vi "Add to data plot.vi"(1 "Data Plot In":T2, 2 "All Data":T1 format="%^_6g", 3 "X-Axis":u32) -> (0 "Data PlotOut":T2)   [LabVIEW 2019]
uses:
  Sub Controls/Data Graph.ctl
  Sub Controls/All Data Array.ctl
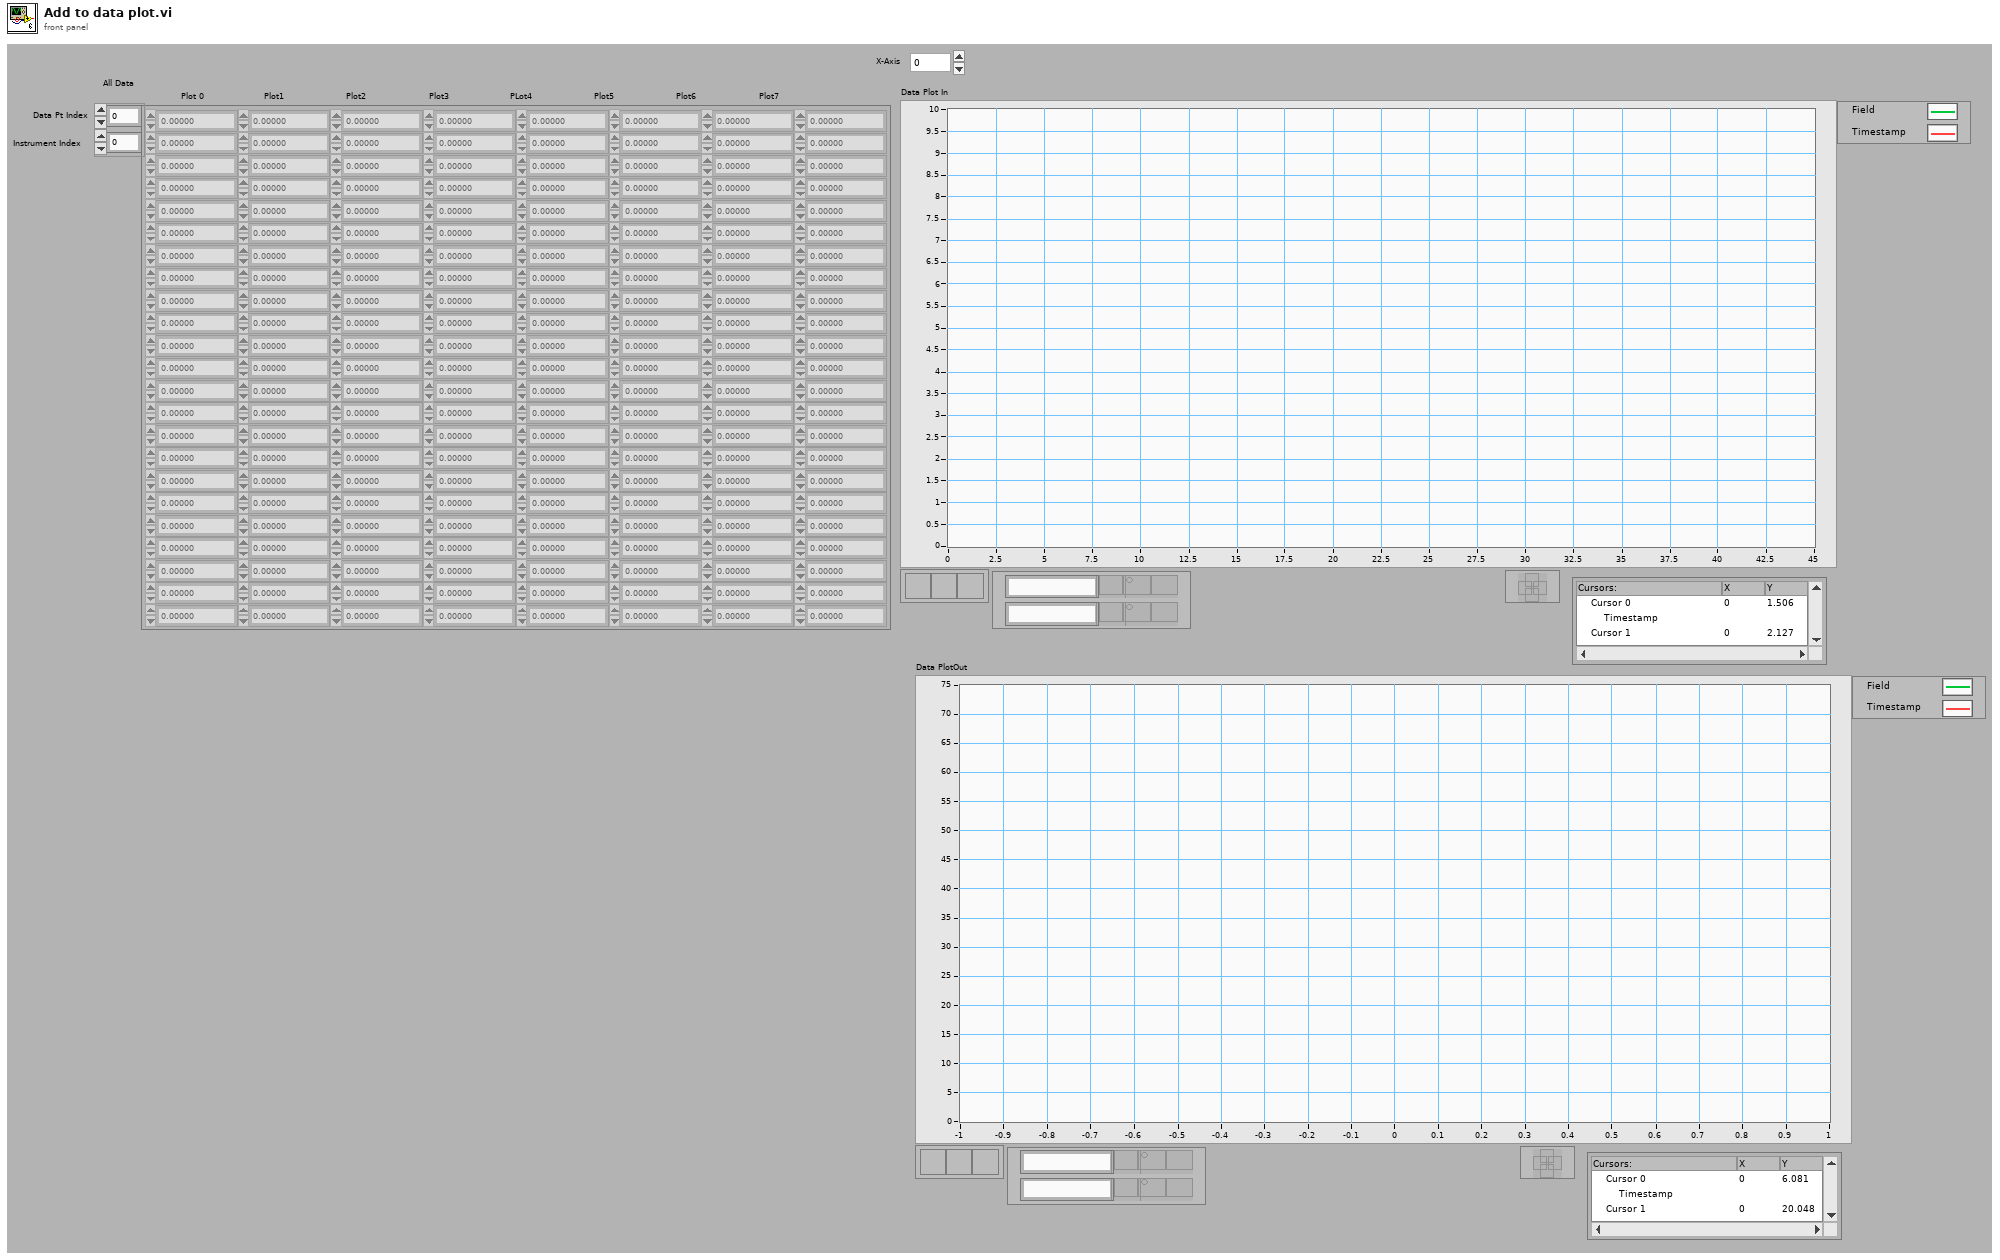
[diagram p1: front panel]
types:
  T1 = typedef "All Data Array.ctl" = dbl[][]
  T2 = typedef "Data Graph.ctl" = cluster{dbl[], dbl[]}[]
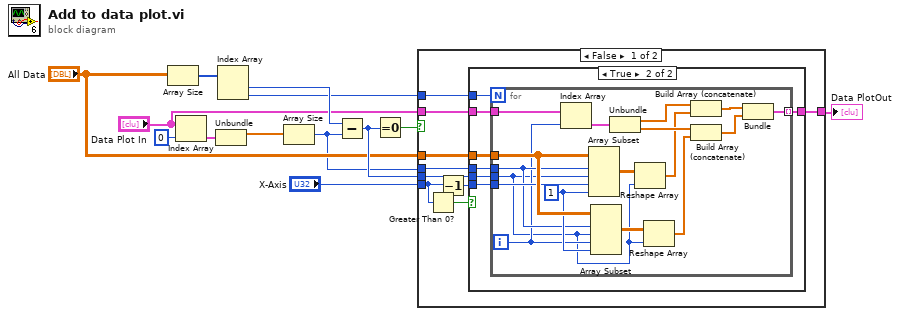
[diagram p0: block diagram]
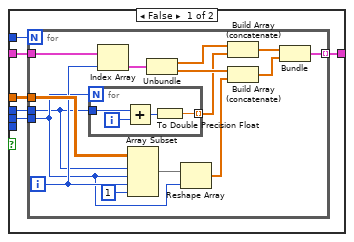
[diagram p2: hidden frame]
diagram:
  n1 = Array Size(array="All Data") -> (size(s)=w10:i32[])
  n2 = Index Array(array="Data Plot In", index=0) -> (element=w9:cluster{dbl[], dbl[]})
  n3 = Unbundle(w9) -> (w8:dbl[])  [unwired: 1 out]
  n4 = Index Array(array=w10) -> (element #1=w11:i32, element #2=w2:i32)  [unwired: 2 in]
  n5 = Array Size(array=w8) -> (size(s)=w4:i32)
  n6 = Subtract(x=w11, y=w4) -> (x-y=w6:i32)
  n7 = Equal To 0?(x=w6) -> (x = 0?=w12:bool)
  n8 = case shown="False" w12 {
    tunnel: [w18 w72] -> w13
    tunnel: "Data Plot In" -> [w22 w72]
    tunnel: w6 -> [w19 _]
    tunnel: "All Data" -> [w21 _]
    tunnel: w4 -> [w20 _]
    tunnel: "X-Axis" -> [w15 _]
    tunnel: w2 -> [w17 _]
    frame False {
      n9 = Greater Than 0?(x=w15) -> (x > 0?=w16:bool)
      n10 = Decrement(x=w15) -> (x-1=w14:u32)
      n11 = case shown="True" w16 {
        tunnel: w22 -> [w23 w54]
        tunnel: w21 -> [w26 w53]
        tunnel: w20 -> [w25 w52]
        tunnel: w19 -> [w24 w51]
        tunnel: [w27 w50] -> w18
        tunnel: w14 -> [_ w49]
        tunnel: w17 -> [w28 w48]
        frame False {
          n12 = for {
            N: w28 -> [_]
            tunnel: w23 -> [w43]
            tunnel: w26 -> [w42]
            tunnel: w25 -> [w30]
            tunnel: w24 -> [w31]
            tunnel: [w40] -> w27 mode=indexing
            i -> [w33]
            n13 = for {
              N: w31 -> [_]
              tunnel: w30 -> [w47]
              tunnel: [w44] -> w29 mode=indexing
              i -> [w46]
              n14 = Add(x=w47, y=w46) -> (x+y=w45:i32)
              n15 = To Double Precision Float(number=w45) -> (double precision float=w44:dbl)
            }
            n16 = Index Array(array=w43, index=w33) -> (element=w34:cluster{dbl[], dbl[]})
            n17 = Array Subset(array=w42, index (row)=w30, length (row)=w31, index (col)=w33, length (col)=1 ("length")) -> (w38:T1)
            n18 = Unbundle(w34) -> (w32:dbl[], w37:dbl[])
            n19 = Reshape Array(w38, w31) -> (w36:dbl[])
            n20 = Build Array (concatenate)(w32, w29) -> (w41:dbl[])
            n21 = Build Array (concatenate)(w37, w36) -> (w39:dbl[])
            n22 = Bundle(w41, w39) -> (w40:cluster{dbl[], dbl[]})  [unwired: 1 in]
          }
        }
        frame True {
          n23 = for {
            N: w48 -> [_]
            tunnel: w54 -> [w71]
            tunnel: w53 -> [w70]
            tunnel: w52 -> [w59]
            tunnel: w51 -> [w55]
            tunnel: [w67] -> w50 mode=indexing
            tunnel: w49 -> [w61]
            i -> [w57]
            w60 = 1 ("length")
            n24 = Index Array(array=w71, index=w57) -> (element=w58:cluster{dbl[], dbl[]})
            n25 = Array Subset(array=w70, index (row)=w59, length (row)=w55, index (col)=w61, length (col)=w60) -> (w69:T1)
            n26 = Array Subset(array=w70, index (row)=w59, length (row)=w55, index (col)=w57, length (col)=w60) -> (w65:T1)
            n27 = Unbundle(w58) -> (w56:dbl[], w64:dbl[])
            n28 = Reshape Array(w69, w55) -> (w63:dbl[])
            n29 = Reshape Array(w65, w55) -> (w62:dbl[])
            n30 = Build Array (concatenate)(w56, w63) -> (w68:dbl[])
            n31 = Build Array (concatenate)(w64, w62) -> (w66:dbl[])
            n32 = Bundle(w68, w66) -> (w67:cluster{dbl[], dbl[]})  [unwired: 1 in]
          }
        }
      }
    }
    frame True {
    }
  }
  "Data PlotOut" <- w13
